vi "Helper VI - DCSM Cut Offs Changed.vi"(7 "New Upper Cut-Off":i32, 9 "Old Lower Cut-Off":i32, 10 "Old Upper Cut-Off":i32, 11 "New Lower Cut-Off":i32) -> (1 "New Lower Cut-Off out":i32, 2 "New Upper Cut-Off out":i32, 3 "Changed?":bool)   [LabVIEW 2023]
doc: "Check to see if the Upper or Lower Cut-Off frequency values have changed since the last iteration."
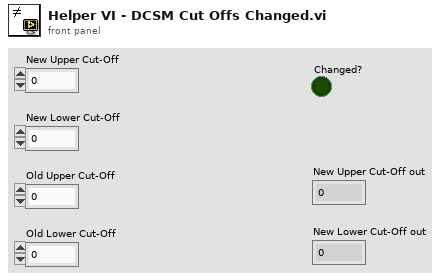
[diagram p1: front panel]
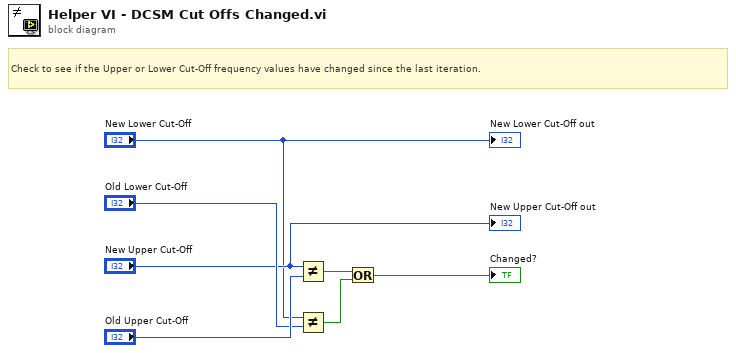
[diagram p0: block diagram]
diagram:
  # "Check to see if the Upper or Lower Cut-Off frequency values have changed since the last iteration."
  n1 = Not Equal?(x="New Upper Cut-Off", y="Old Upper Cut-Off") -> (x != y?=w7:bool)
  n2 = Not Equal?(x="New Lower Cut-Off", y="Old Lower Cut-Off") -> (x != y?=w6:bool)
  n3 = Or(x=w7, y=w6) -> (x .or. y?=→"Changed?":bool)
  "New Lower Cut-Off out" <- "New Lower Cut-Off"
  "New Upper Cut-Off out" <- "New Upper Cut-Off"
